vi "identify new classes.vi"(8 "error in":errorcluster, 10 "force scan":bool, 11 "cache in":T1) -> (0 "error out":errorcluster, 3 "cache out":T1)   [LabVIEW 2013, in "PL_class cache.lvlib"]
uses:
  PL_class cache.lvlib
  cache definition.ctl
  cache search configuration.ctl
  cached class information.ctl
  target class metadata.ctl
  class metadata.ctl
  <vilib>/NI/Tag Bus Module Framework/root configuration/Target Types.ctl
  <vilib>/NI/CEF/CEF_TreeControl/class discovery singleton/class discovery singleton methods.ctl
  cache data.vi
  <vilib>/NI/CEF/CEF_TreeControl/class discovery singleton/class discovery singleton.lvlib
  <vilib>/NI/Tag Bus Module Framework/root configuration/TBM configuration.lvclass
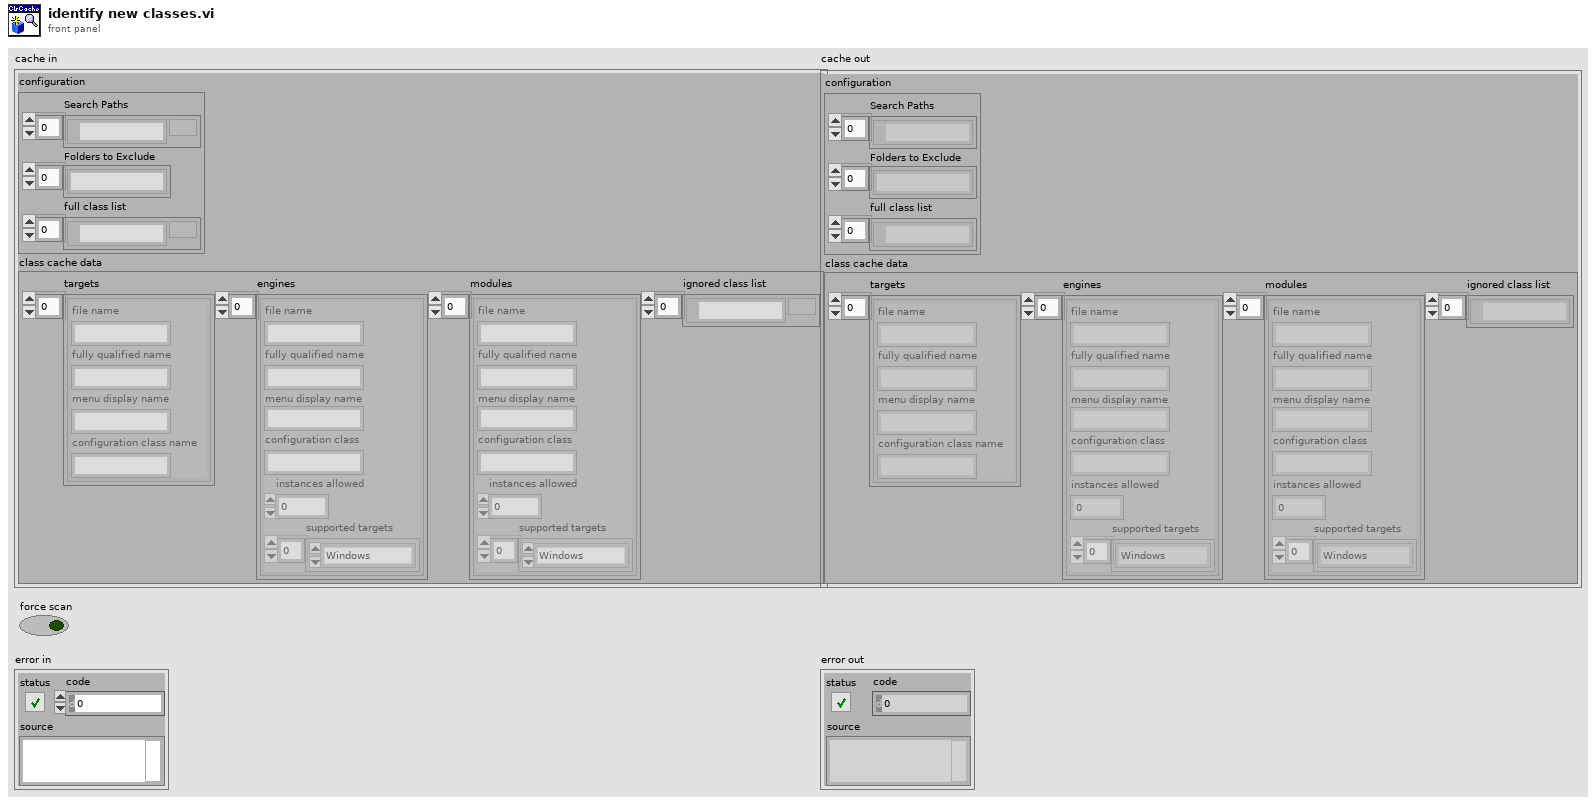
[diagram p1: front panel]
types:
  T1 = typedef "PL_class cache.lvlib/cache definition.ctl" = cluster{"configuration":T2, "class cache data":T3}
  T2 = typedef "PL_class cache.lvlib/cache search configuration.ctl" = cluster{"Search Paths":path[], "Folders to Exclude":string[], "full class list":path[]}
  T3 = typedef "PL_class cache.lvlib/cached class information.ctl" = cluster{"targets":T4[], "engines":T5[], "modules":T5[], "ignored class list":path[]}
  T4 = typedef "PL_class cache.lvlib/target class metadata.ctl" = cluster{"file name":string, "fully qualified name":string, "menu display name":string, "configuration class name":string}
  T5 = typedef "PL_class cache.lvlib/class metadata.ctl" = cluster{"file name":string, "fully qualified name":string, "menu display name":string, "configuration class":string, "instances allowed":i32, "supported targets":T6[]}
  T6 = typedef "TBM configuration.lvclass/Target Types.ctl" = enum16{"Windows", "Mac", "Linux", "Linux RT ARM", "VxWorks", "Pharlap", "Other", "Linux RT x64"}
  T7 = typedef "class discovery singleton.lvlib/class discovery singleton methods.ctl" = enum16{"add search paths", "load class by name", "list available classes", "get class path"}
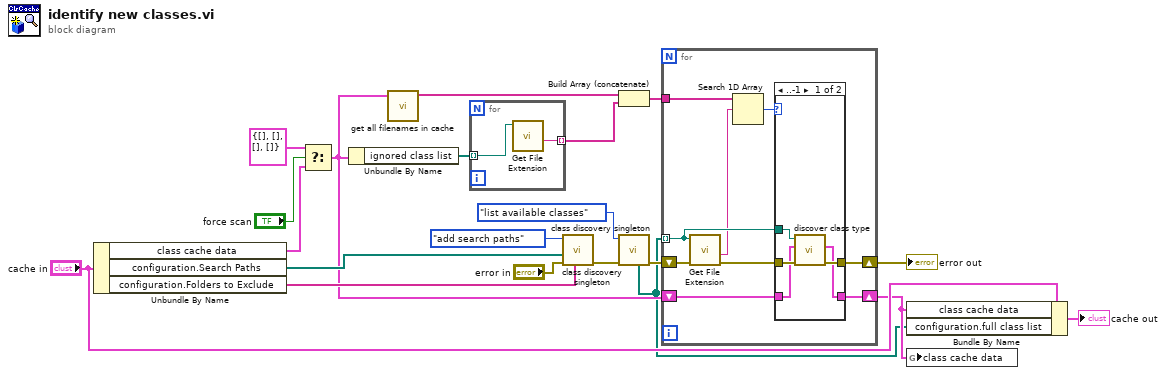
[diagram p0: block diagram]
diagram:
  n1 = Unbundle By Name("cache in") -> ("class cache data"=w16:T3, "configuration.Search Paths"=w13:path[], "configuration.Folders to Exclude"=w12:string[])
  n2 = Select(t=T3 {"targets"=[], "engines"=[], "modules"=[], "ignored class list"=[]} ("class cache data"), s="force scan", f=w16) -> (s? t:f=w5:T3)
  n3 = Unbundle By Name(w5) -> ("ignored class list"=w4:path[])
  n4 = call "get all filenames in cache.vi"("class cache data"=w5) -> ("Array"=w7:string[])  [unwired: 10 in]
  n5 = for {
    tunnel: [w22] -> w2 mode=indexing
    tunnel: w4 -> [w21] mode=indexing
    n6 = call <vilib>:"Get File Extension.vi"("file"=w21) -> ("filename without extension"=w22:string)  [unwired: 7 in, 3 out]
  }
  n7 = call <vilib>:"class discovery singleton.vi"("Folders to Exclude"=w12, "error in"="error in", "Plugin Search Paths"=w13, "method"=class_discovery_singleton_methods."add search paths") -> ("error out"=w11:errorcluster)  [unwired: 4 in, 3 out]
  n8 = Build Array (concatenate)(w7, w2) -> (w3:string[])
  n9 = call <vilib>:"class discovery singleton.vi"("error in"=w11, "method"=class_discovery_singleton_methods."list available classes") -> ("error out"=w10:errorcluster, "discovered classes"=w1:path[])  [unwired: 6 in, 2 out]
  n10 = for {
    tunnel: w1 -> [w26] mode=indexing
    shift-right: [w31] -> w6
    shift-left: w5 -> [w30]
    shift-right: [w29] -> w17
    shift-left: w10 -> [w28]
    tunnel: w3 -> [w25]
    n11 = call <vilib>:"Get File Extension.vi"("error in (no error)"=w28, "file"=w26) -> ("error out"=w27:errorcluster, "filename without extension"=w24:string)  [unwired: 6 in, 2 out]
    n12 = Search 1D Array(1D array=w25, element=w24) -> (index of element=w23:i32)  [unwired: 1 in]
    n13 = case shown="..-1" w23 {
      tunnel: [w32 w38] -> w31
      tunnel: w30 -> [w33 w38]
      tunnel: [w34 w37] -> w29
      tunnel: w27 -> [w36 w37]
      tunnel: w26 -> [w35 _]
      frame ..-1 {
        n14 = call "discover class type.vi"("error in"=w36, "class cache data in"=w33, "Path"=w35) -> ("error out"=w34:errorcluster, "class cache data out"=w32:T3)  [unwired: 7 in]
      }
      frame 0.. {
      }
    }
  }
  "error out" <- w17
  n15 = Bundle By Name(cluster="cache in", "class cache data"=w6, "configuration.full class list"=w1) -> (→"cache out":T1)
  n16 = global write "cache data.vi" "class cache data"(w6) -> ()
